vi "keynav_keybinds.vi"(1 "Key":T1(ring)) -> (0 "Tab id":i32)   [LabVIEW 2017]
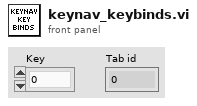
[diagram p1: front panel]
types:
  T1 = enum16{"0", "1", "2", "3", "4", "5", "6", "7", "8", "9", "A", "B", "C", "D", "E", "F", "G", "H", "I", "J", "K", "L", "M", "N", "O", "P", "Q", "R", "S", "T", "U", "V", "W", "X", "Y", "Z", "F1", "F2", "F3", "F4", "F5", "F6", "F7", "F8", "F9", "F10", "F11", "F12", "F13", "F14", "F15", "ADD", "BACK", "BACKSLASH", "CAPITAL", "COMMA", "DECIMAL", "DELETE", "DIVIDE", "DOWN", "END", "EQUALS", "ESCAPE", "GRAVE (`)", "HOME", "INSERT", "LBRACKET", "LCONTROL", "LEFT", "L ALT", "LSHIFT", "LWIN", "MINUS", "MULTIPLY", "NEXT", "NUMLOCK", "NUMPAD_0", "NUMPAD_1", "NUMPAD_2", "NUMPAD_3", "NUMPAD_4", "NUMPAD_5", "NUMPAD_6", "NUMPAD_7", "NUMPAD_8", "NUMPAD_9", "PAUSE", "PERIOD", "PRIOR (PG UP)", "RBRACKET", "RCONTROL", "RETURN", "RIGHT", "R ALT", "RSHIFT", "RWIN", "SCROLL", "SEMICOLON", "SLASH", "SPACE", "SUBTRACT", "TAB", "UP", "ENTER (num pad)", "' (quote)"}
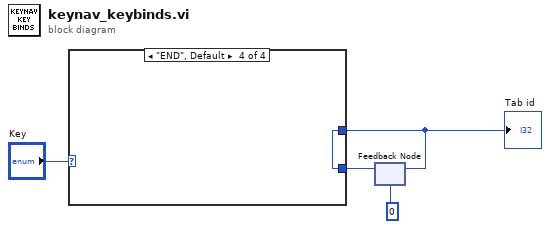
[diagram p0: block diagram]
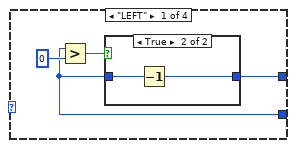
[diagram p2: hidden frame]
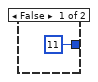
[diagram p3: hidden frame]
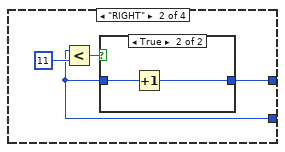
[diagram p4: hidden frame]
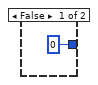
[diagram p5: hidden frame]
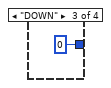
[diagram p6: hidden frame]
diagram:
  n1 = feedback #1(0) -> (w2:i32)
  n2 = case shown="\"END\", Default" "Key" {
    tunnel: w2 -> [w6 w13 _ w20]
    tunnel: [w5 w12 0 w20] -> w4
    frame "LEFT" {
      n3 = Greater?(x=w6, y=0) -> (0:w8:bool)
      n4 = case shown="True" w8 {
        tunnel: w6 -> [_ w11]
        tunnel: [11 w10] -> w5
        frame False {
        }
        frame True {
          n5 = Decrement(x=w11) -> (x-1=w10:i32)
        }
      }
    }
    frame "RIGHT" {
      n6 = Less?(x=w13, y=11) -> (x < y?=w15:bool)
      n7 = case shown="True" w15 {
        tunnel: w13 -> [_ w18]
        tunnel: [0 w17] -> w12
        frame False {
        }
        frame True {
          n8 = Increment(x=w18) -> (x+1=w17:i32)
        }
      }
    }
    frame "DOWN" {
    }
    frame "END", Default {
    }
  }
  "Tab id" <- w4
  n9 = feedback-in #1(w4) -> ()
